vi "Write 2D Array of Double To XL.vi"(8 "error in":errorcluster, 10 "Write/Read Cell Numeric":T1 {"Data 1D" format="%.2f"; "Data 2D" format="%.2f"; "1 Data" format="%.2f"}, 11 "Work Sheet":refnum<k7>) -> (0 "error out":errorcluster, 3 "Work Sheet":refnum<k7>)   [LabVIEW 2017]
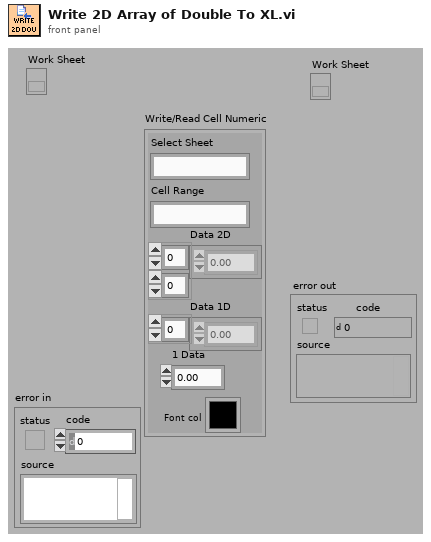
[diagram p1: front panel]
types:
  T1 = cluster{"Cell Range":string, "Select Sheet":string, "1 Data":dbl, "Data 2D":dbl[][], "Data 1D":dbl[], "Font col":u32}
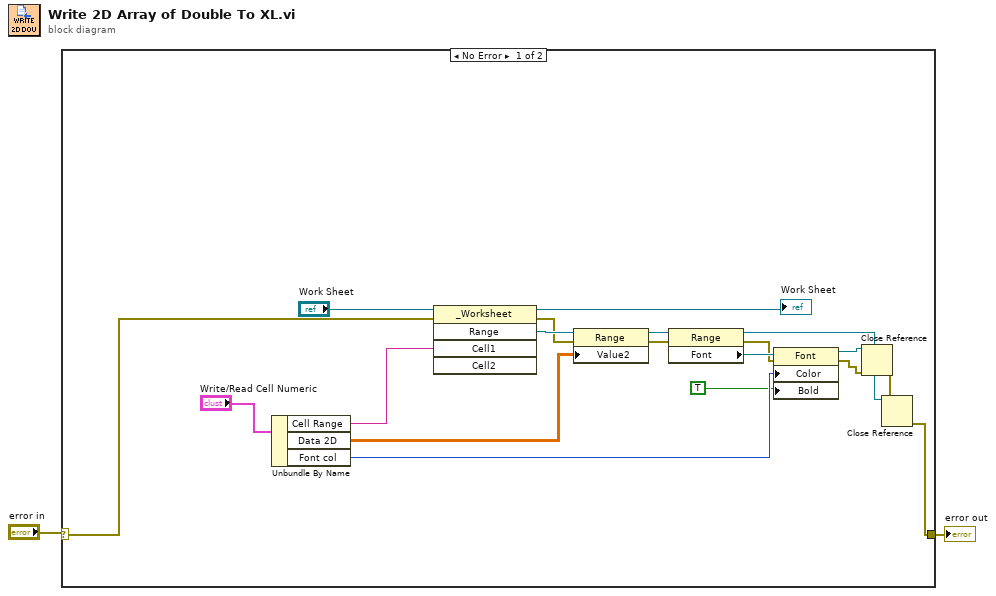
[diagram p0: block diagram]
diagram:
  n1 = case shown="No Error" "error in" {
    selector: "error in" -> [w20 w22]
    tunnel: [w6 w22] -> w1
    frame No Error {
      n2 = Unbundle By Name("Write/Read Cell Numeric") -> ("Cell Range"=w15:string, "Data 2D"=w16:dbl[][], "Font col"=w11:u32)
      n3 = invoke class="_Worksheet" method="Range"(reference="Work Sheet", error in=w20, "Cell1"=w15) -> (reference out=→"Work Sheet":refnum<k7>, error out=w19:errorcluster, "Range"=w21:refnum<k7>)  [unwired: 2 in, 2 out]
      n4 = property class="Range"(reference=w21, error in=w19, "Value2"=w16) -> (reference out=w13:refnum<k7>, error out=w5:errorcluster)
      n5 = property class="Range"(reference=w13, error in=w5) -> (reference out=w8:refnum<k7>, error out=w4:errorcluster, "Font"=w12:refnum<k7>)
      n6 = property class="Font"(reference=w12, error in=w4, "Color"=w11, "Bold"=TRUE) -> (reference out=w10:refnum<k7>, error out=w9:errorcluster)
      n7 = Close Reference(reference=w10, error in (no error)=w9) -> (error out=w7:errorcluster)
      n8 = Close Reference(reference=w8, error in (no error)=w7) -> (error out=w6:errorcluster)
    }
    frame Error {
    }
  }
  "error out" <- w1
